vi "TimeSampleDlgModify.vi"(10 "序号":string, 11 "定时采样信息in":T1) -> (2 "定时采样信息":T1)   [LabVIEW 2014, in "Sample.lvlib"]
uses:
  Sample.lvlib
  DataBase/DataBase.lvlib
panel:
  in  "备注":string
  out "电压范围":string
  in  "取消按钮":bool
  in  "确定按钮":bool
  in  "电源频率（Hz）":string="1"
  in  "电源电压":string
  in  "分钟":u16(ring) items=["0", "01", "02", "03", "04", "05", "06", "07", "08", "09", "10", "11", "12", "13", "14", "15", "16", "17", "18", "19", "20", "21", "22", "23", "24", "25", "26", "27", "28", "29", "30", "31", "32", "33", "34", "35", "36", "37", "38", "39", "40", "41", "42", "43", "44", "45", "46", "47", "48", "49", "50", "51", "52", "53", "54", "55", "56", "57", "58", "59"]
  in  "时":u16(ring) items=["1", "2", "3", "4", "5", "6", "7", "8", "9", "10", "11", "12", "13", "14", "15", "16", "17", "18", "19", "20", "21", "22", "23", "24"]
  in  "检测区域":string(combo)
  in  "是否启动":string(combo)="是"
  in  "检测位置":string(combo)="上层膜检测"
  in  "OK":bool
  # "检测时间"
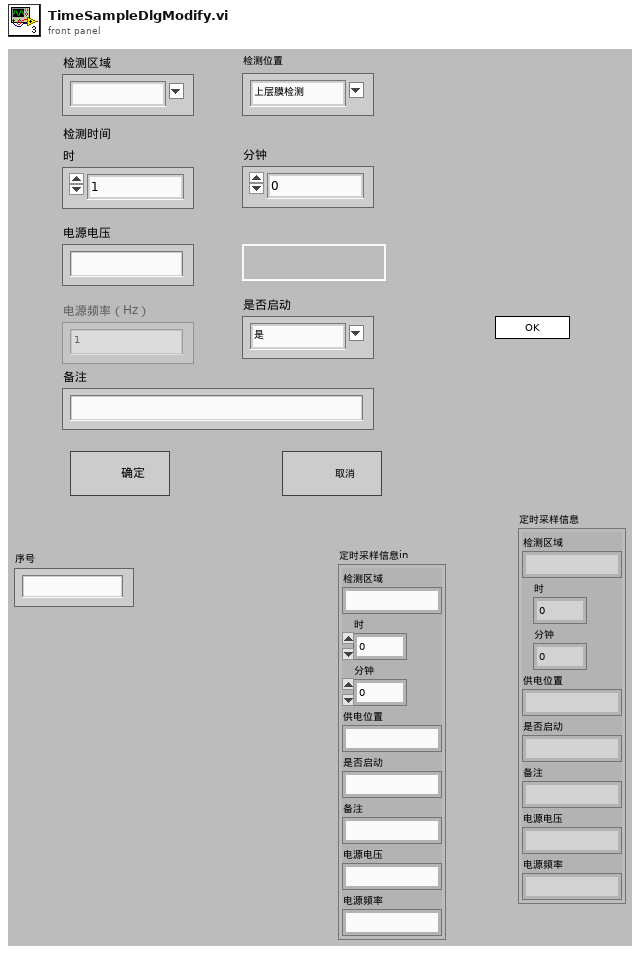
[diagram p1: front panel]
types:
  T1 = cluster{"检测区域":string, "时":u16, "分钟":u16, "供电位置":string, "是否启动":string, "备注":string, "电源电压":string, "电源频率":string}
  T2 = enum32{"invalid app kind", "Development System", "Run Time System", "Student Edition", "Embedded LabVIEW", "Evaluation", "Custom"}
  T3 = enum32{"Invalid", "Standard", "Closed", "Hidden", "Minimized", "Maximized"}
  T4 = cluster{"Core":cluster{"Current VI Reference":refnum<vi>, "Close Panel on Exit?":bool}, "Your Boolean data":bool, "序号":string, "AreaName":string, "SampleAreaName":string[], "定时采样信息":cluster{"检测区域":string, "时":u16, "分钟":u16, "供电位置":string, "是否启动":string, "备注":string, "电源电压":string, "电源频率":string}, "电源倍数":string, "最大电压值":i32, "定时采样info":cluster{"检测区域":string, "时":u16, "分钟":u16, "供电位置":string, "是否启动":string, "备注":string, "电源电压":string, "电源频率":string}}
  T5 = cluster{"Current VI Reference":refnum<vi>, "Close Panel on Exit?":bool}
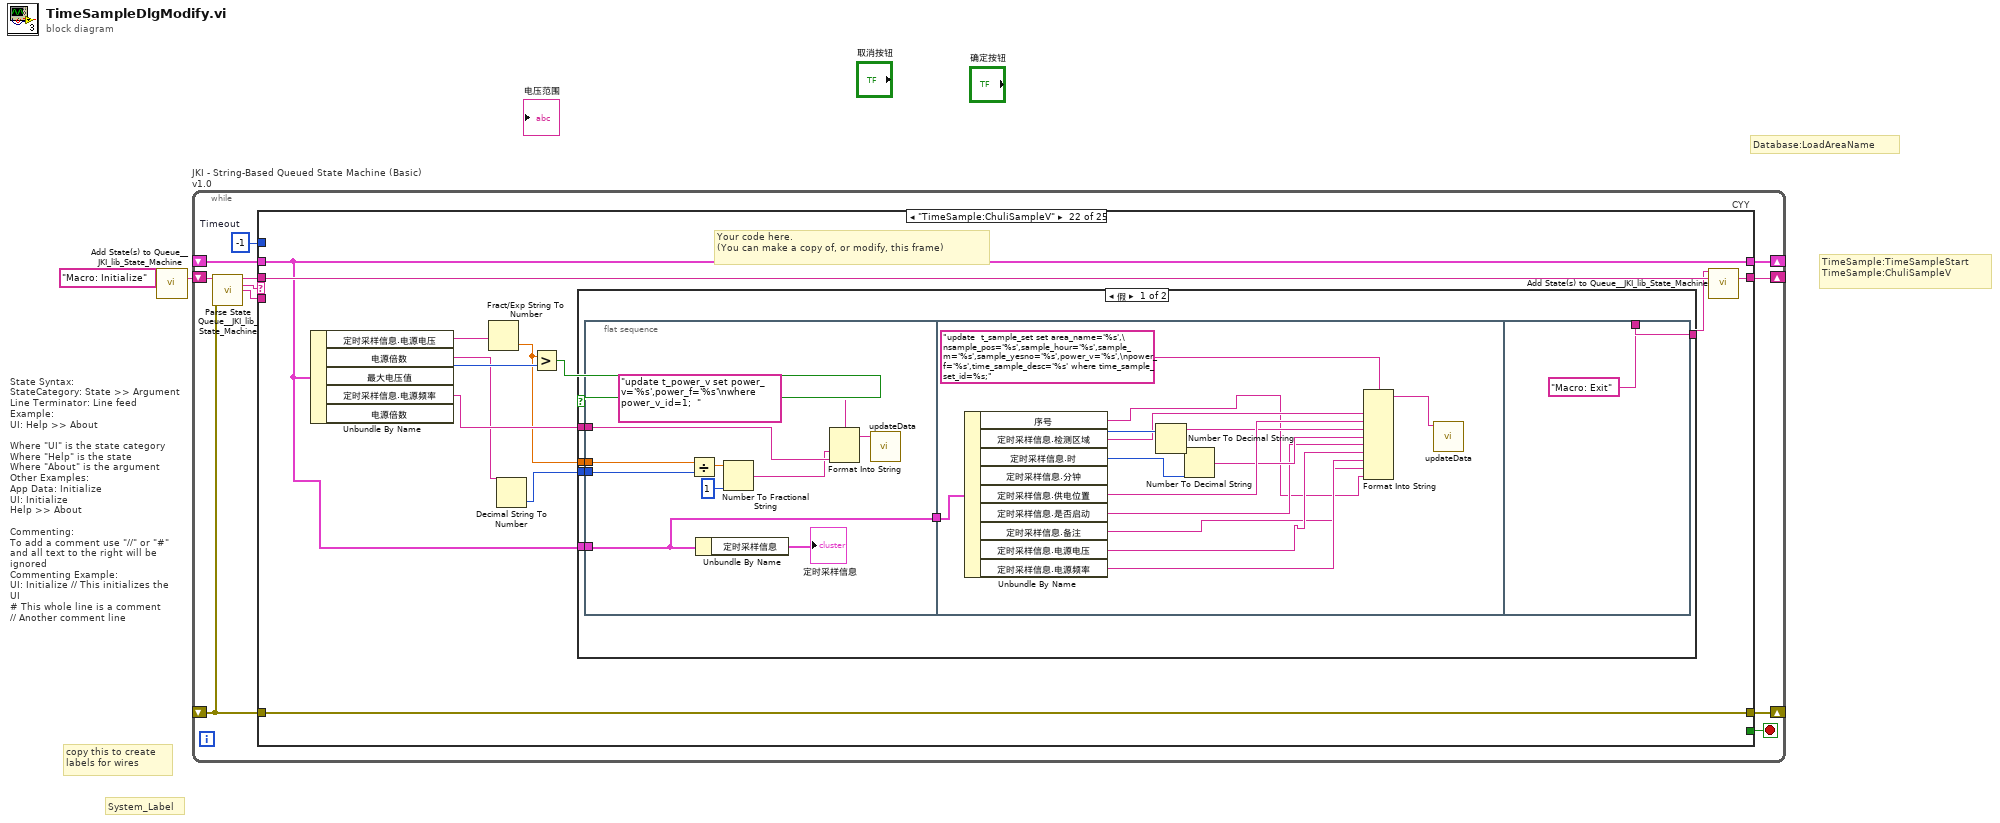
[diagram p0: block diagram]
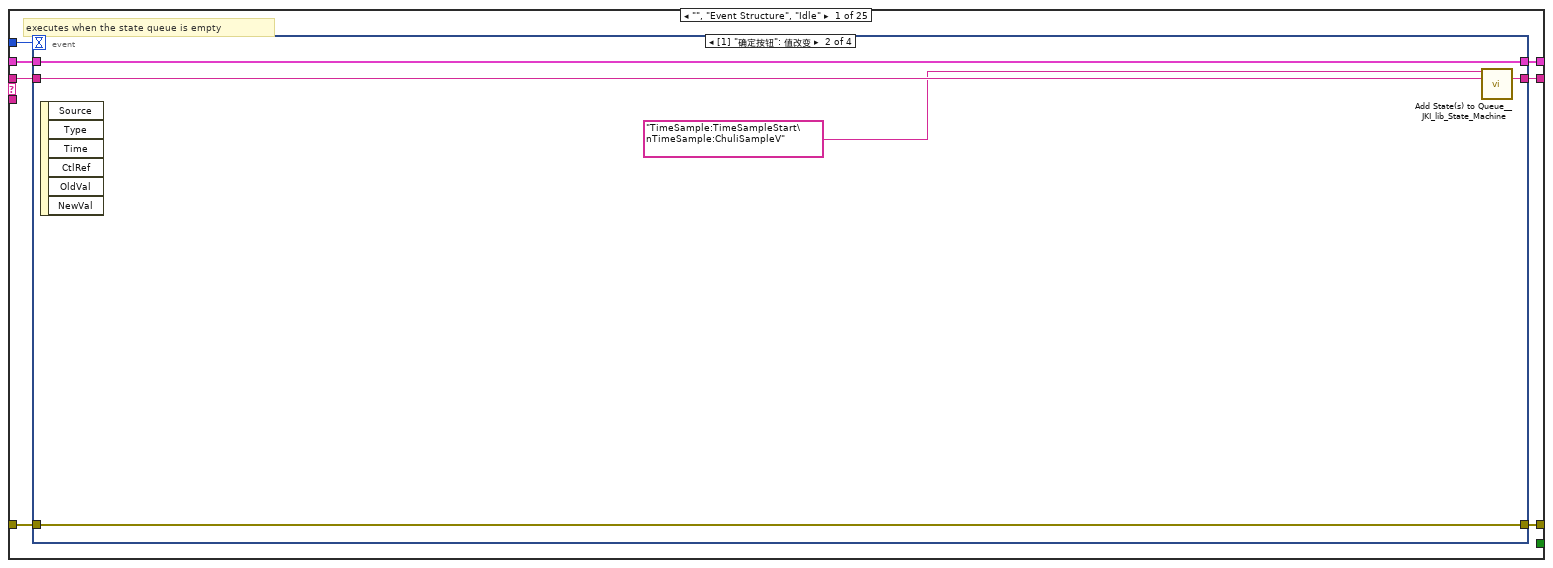
[diagram p2: hidden frame]
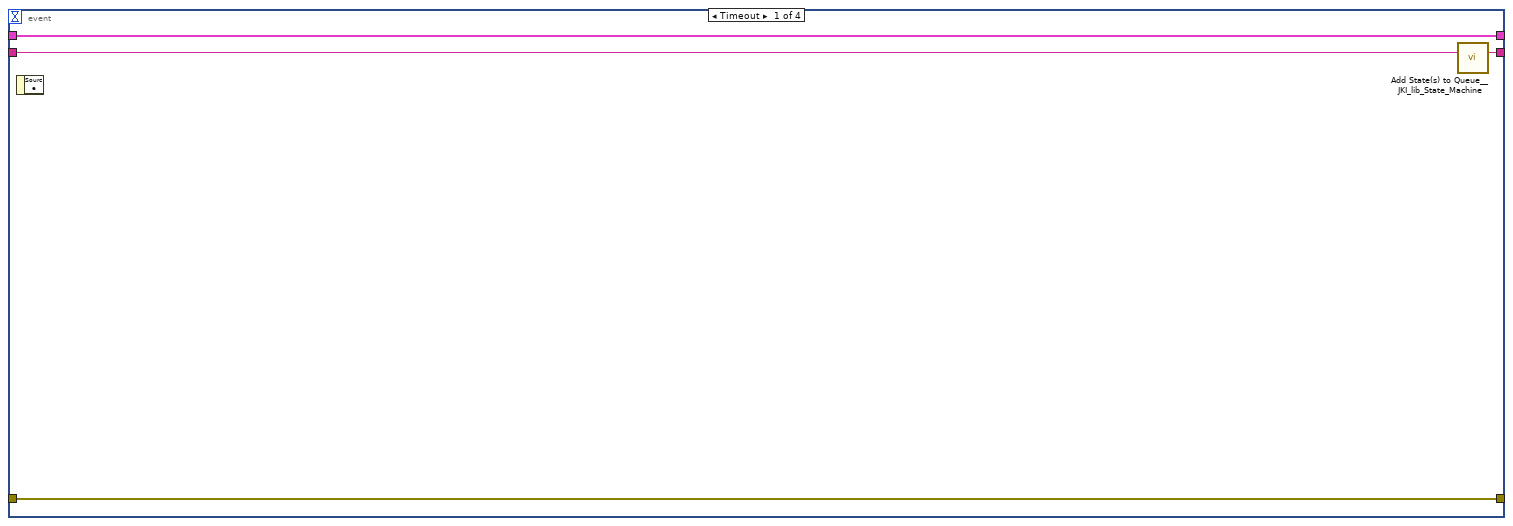
[diagram p3: hidden frame]
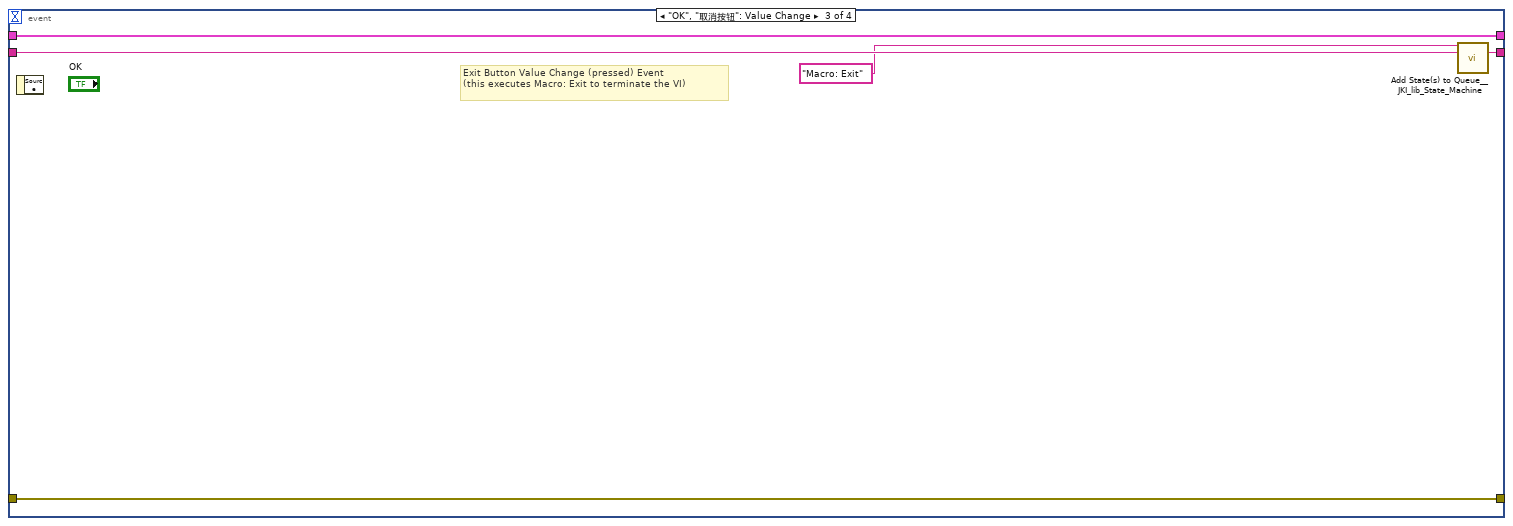
[diagram p4: hidden frame]
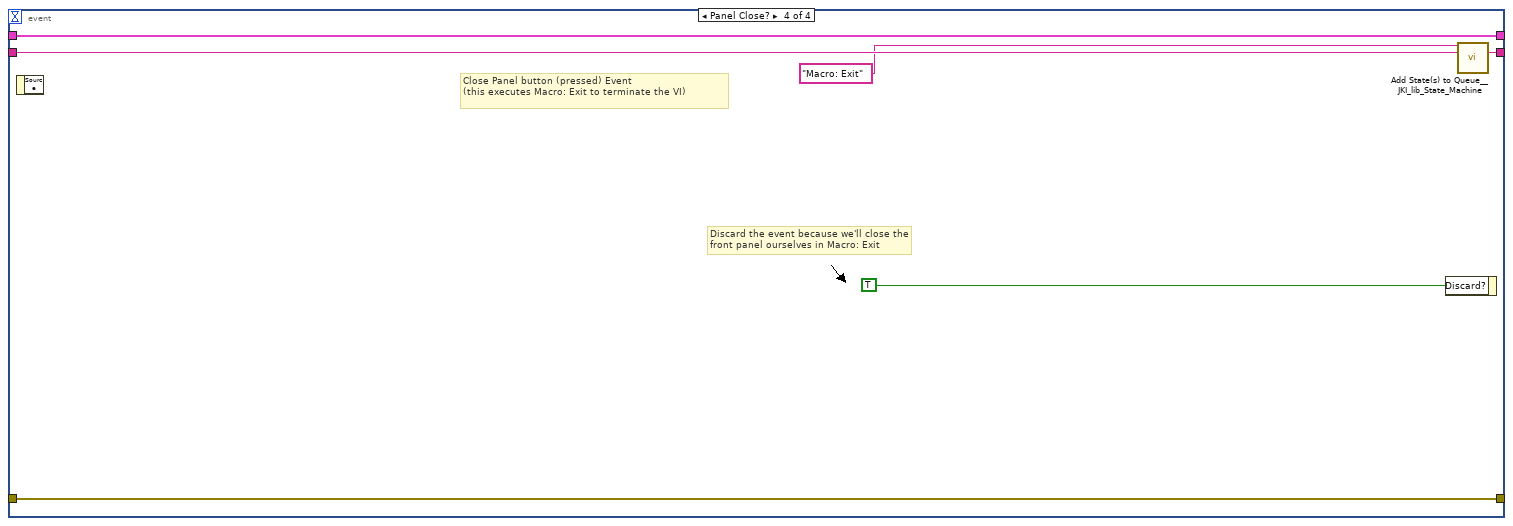
[diagram p5: hidden frame]
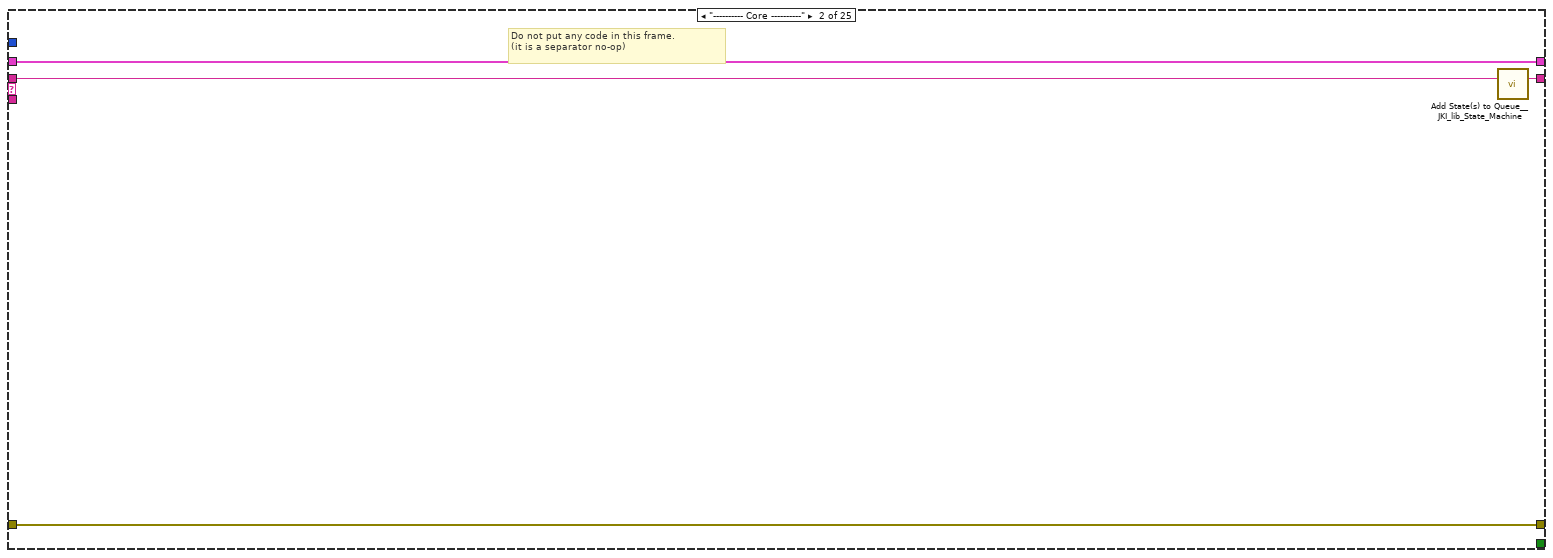
[diagram p6: hidden frame]
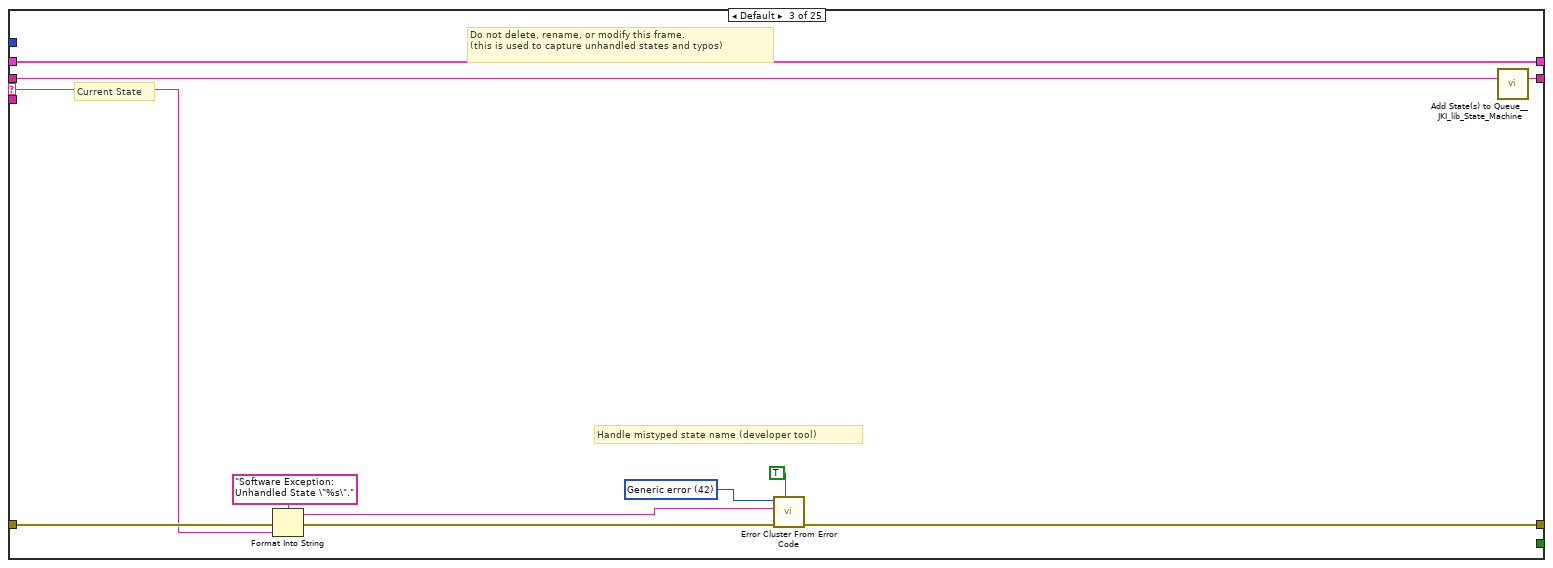
[diagram p7: hidden frame]
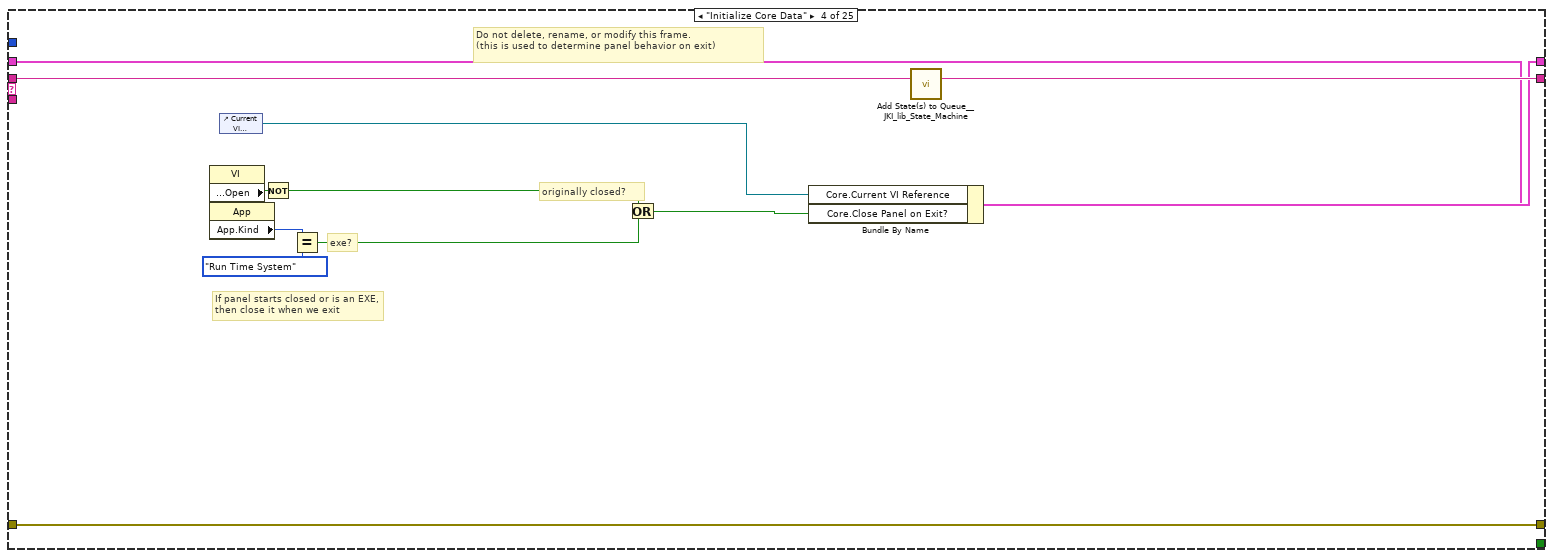
[diagram p8: hidden frame]
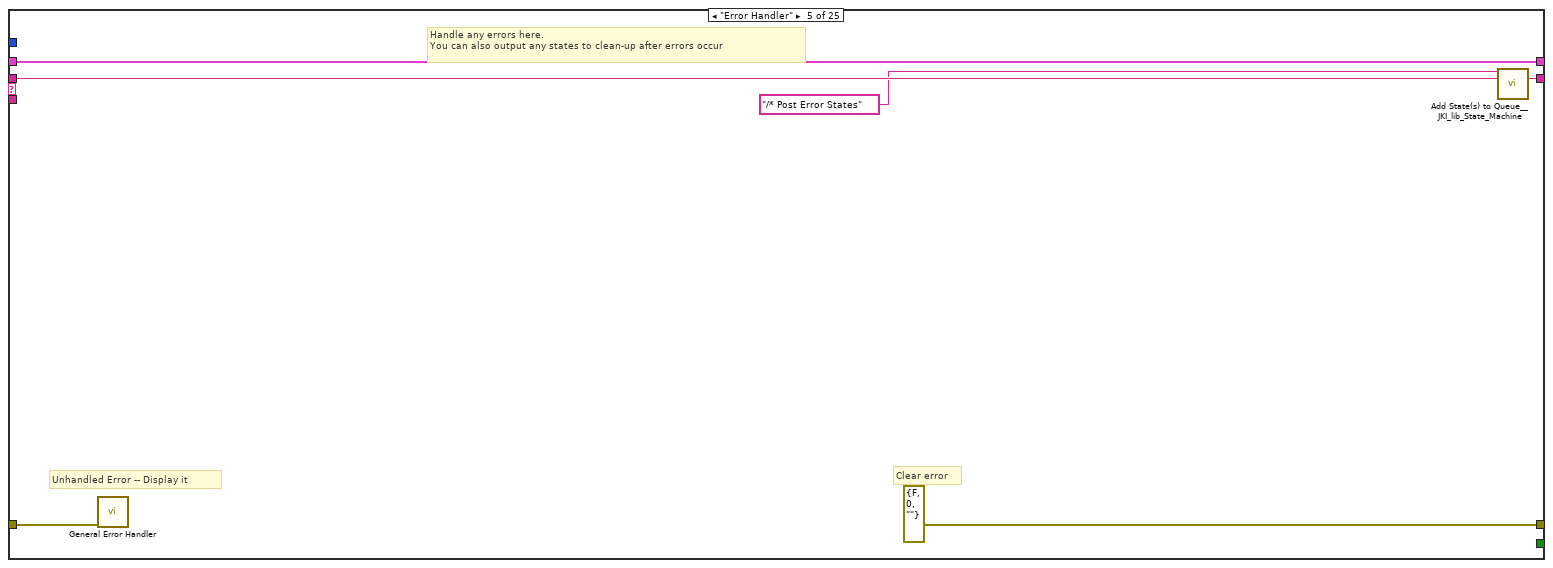
[diagram p9: hidden frame]
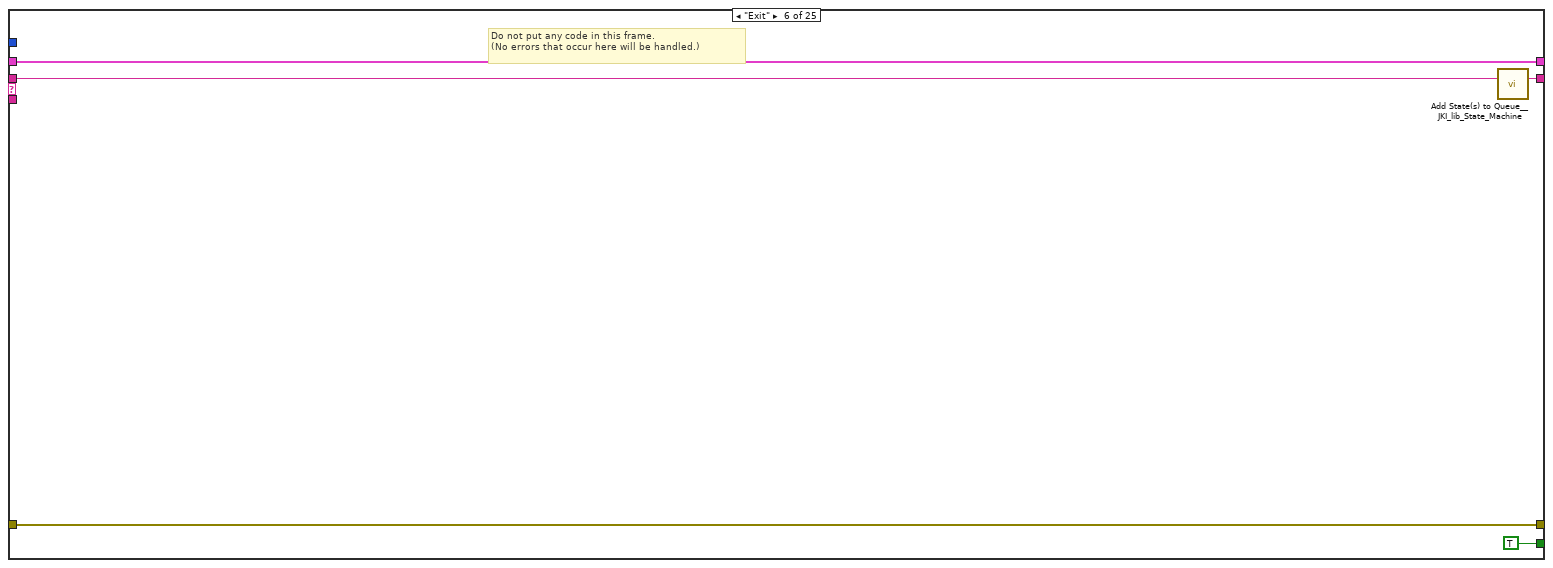
[diagram p10: hidden frame]
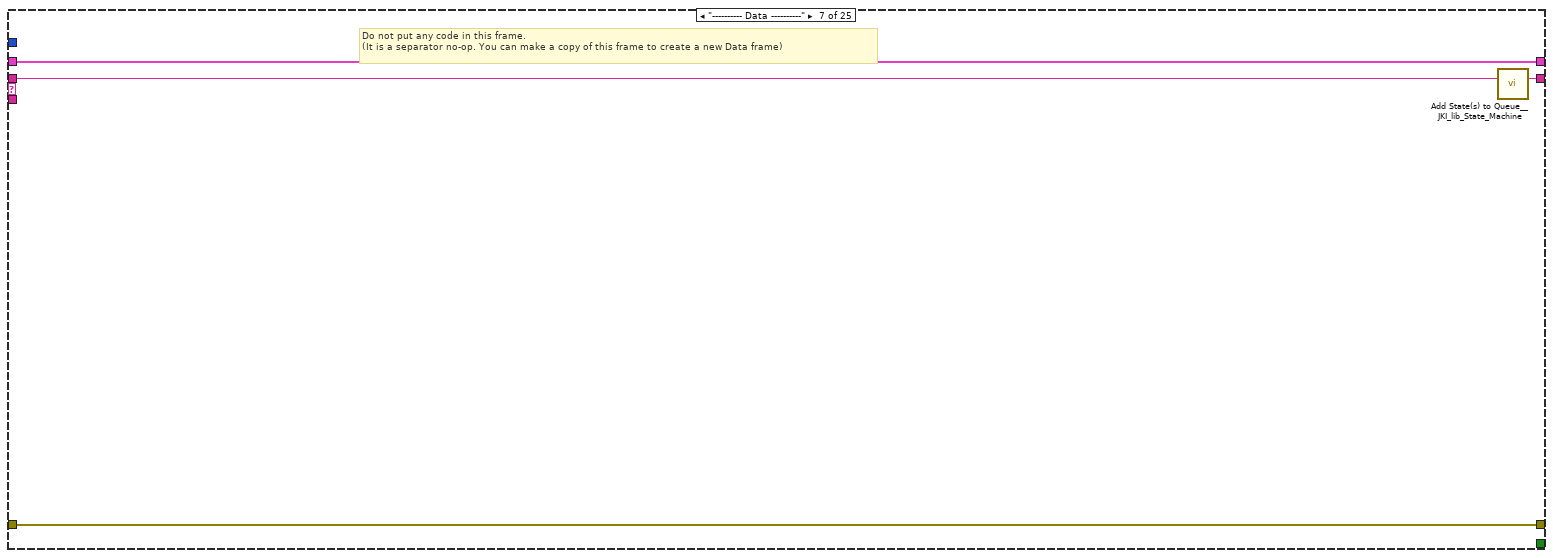
[diagram p11: hidden frame]
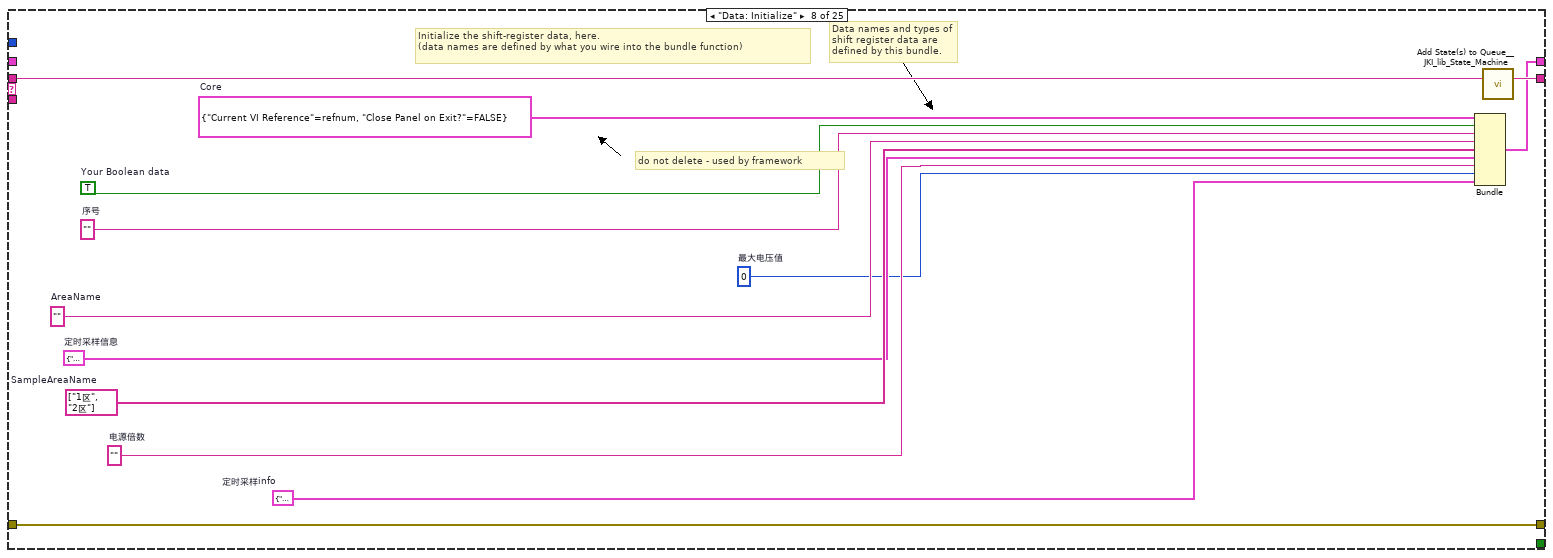
[diagram p12: hidden frame]
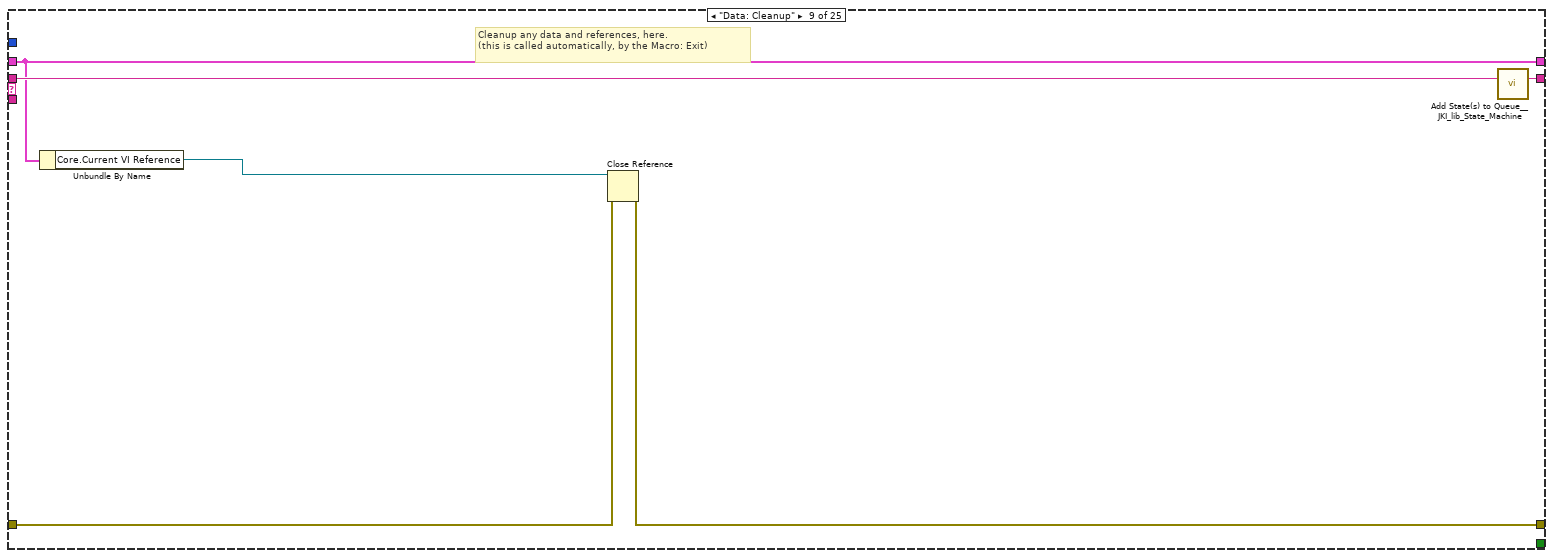
[diagram p13: hidden frame]
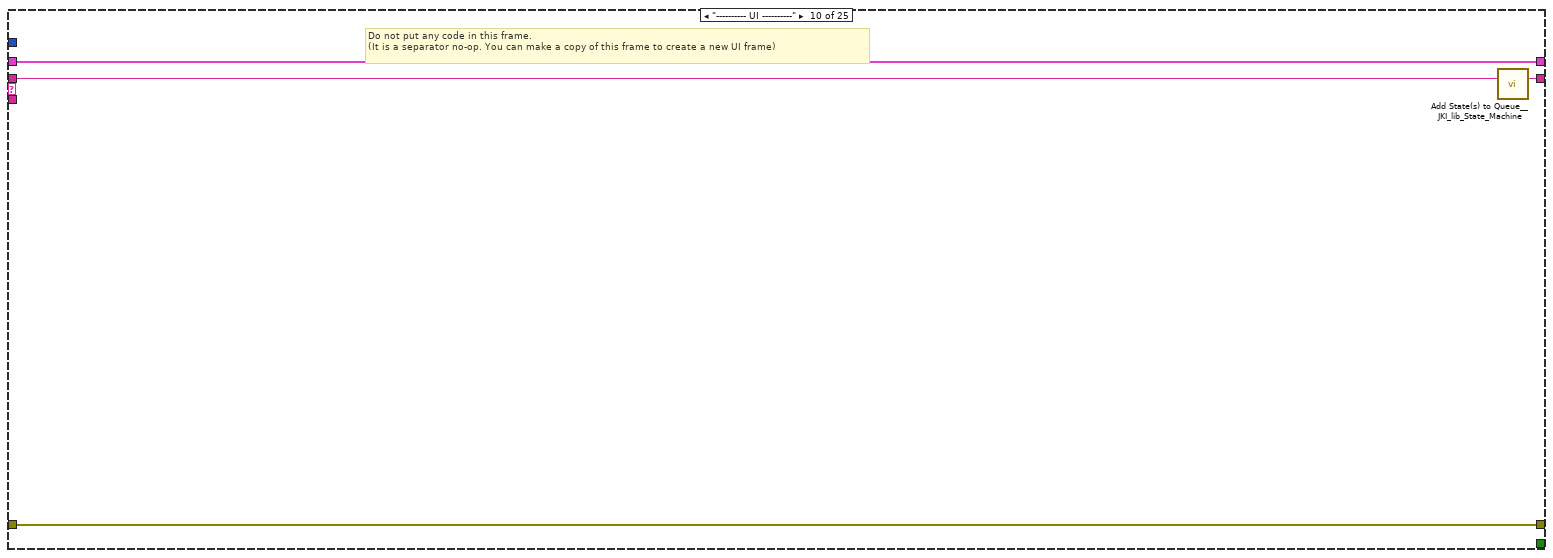
[diagram p14: hidden frame]
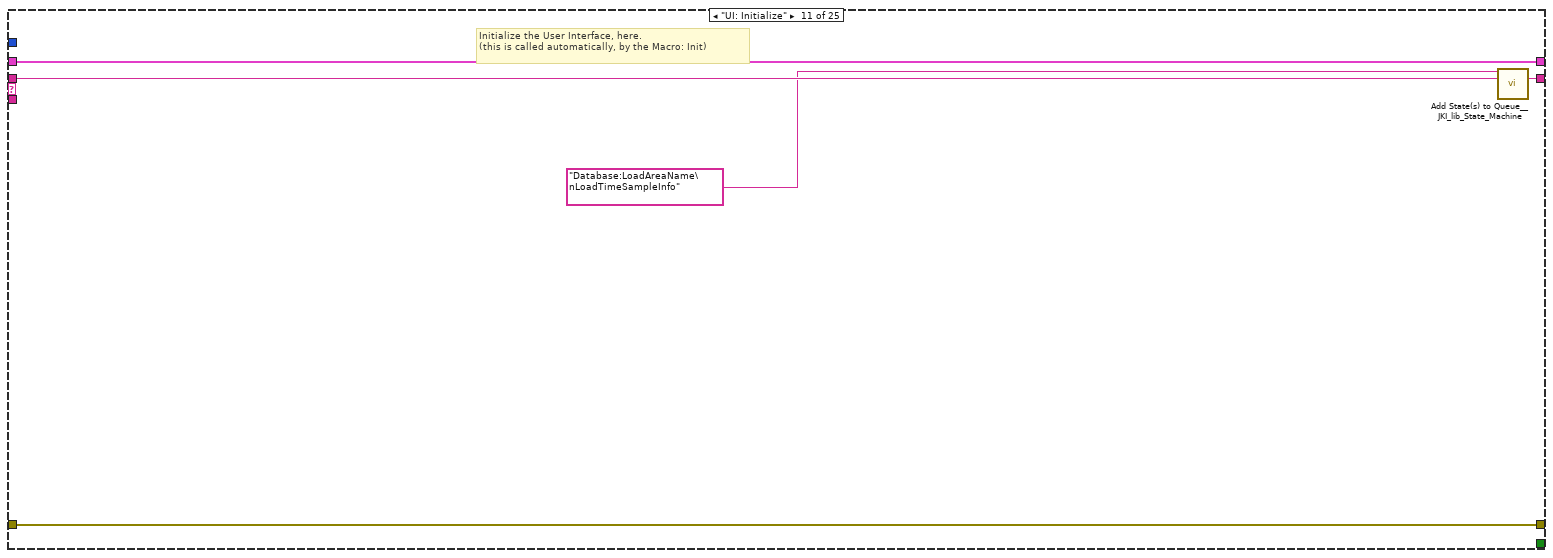
[diagram p15: hidden frame]
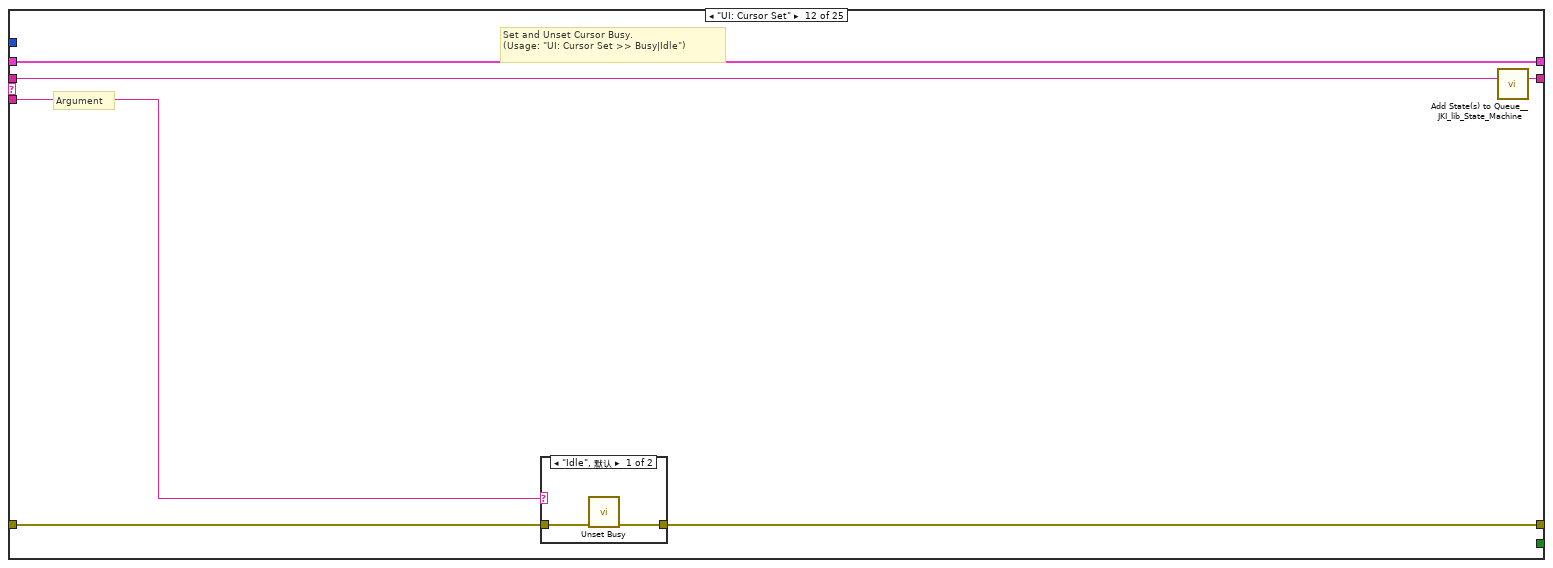
[diagram p16: hidden frame]
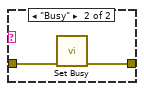
[diagram p17: hidden frame]
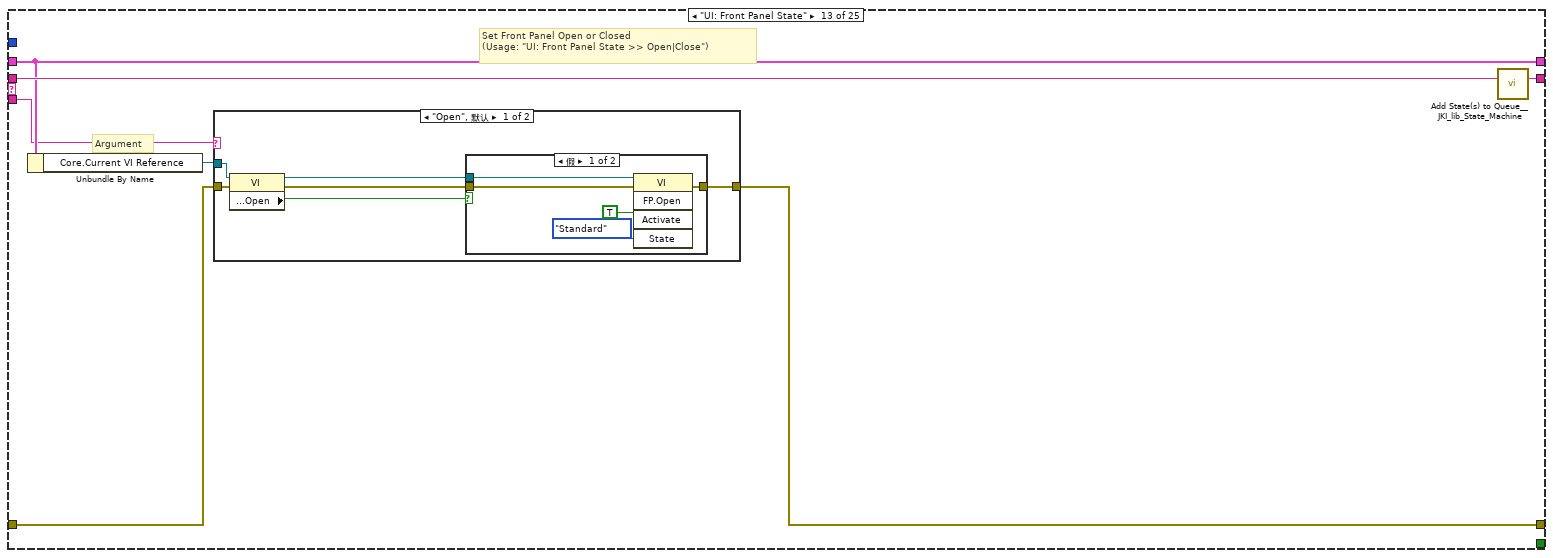
[diagram p18: hidden frame]
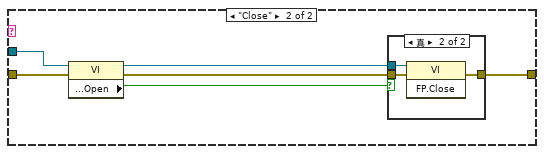
[diagram p20: hidden frame]
diagram:
  # "TimeSample:TimeSampleStart\nTimeSample:ChuliSampleV"
  # "Database:LoadAreaName"
  # "State Syntax:\nStateCategory: State >> Argument\nLine Terminator: Line feed\nExample:\nUI: Help >> About\n\nWhere \"UI\" is the state category\nWhere \"Help\" is the state\nWhere \"About\" is the argument\nOther Examples:\nApp Data: Initialize\nUI: Initialize\nHelp >> About\n\nCommenting:\nTo add a comment use \"//\" or \"#\" and all text to the right will be ignored\nCommenting Example:\nUI: Initialize // This initializes the UI\n# This whole line is a comment\n// Another comment line"
  # "copy this to create labels for wires"
  # "System_Label"
  n1 = call <vilib>:"Add State(s) to Queue__JKI_lib_State_Machine.vi"("State(s) in (\"\")"="Macro: Initialize") -> ("States Out"=w2:string)  [unwired: 14 in]
  n2 = while "JKI - String-Based Queued State Machine (Basic) v1.0" {
    shift-right: [w6] -> _
    shift-left: _ -> [w5]
    shift-right: [w9] -> _
    shift-left: _ -> [w3]
    shift-right: [w8] -> _
    shift-left: w2 -> [w10]
    stop <- w7 stop-if-true
    w4 = -1  # Timeout
    # "CYY"
    n3 = call <vilib>:"Parse State Queue__JKI_lib_State_Machine.vi"("State Queue"=w10, "Error In (no error)"=w3) -> ("Remaining States"=w12:string, "Current State"=w13:string, "Arguments"=w11:string)  [unwired: 11 in]
    n4 = case shown="\"TimeSample:ChuliSampleV\"" w13 {
      selector: w13 -> [_ _ w45 _ _ _ _ _ _ _ _ _ _ _ _ _ _ _ _ _ _ _ _ _ _]
      tunnel: w12 -> [w20 w44 w49 w67 w73 w78 w82 w95 w101 w105 w110 w116 w127 w153 w158 w168 w172 w176 w180 w196 w200 w212 w259 w263 w273]
      tunnel: w11 -> [_ _ _ _ _ _ _ _ _ _ _ w111 w121 _ _ _ _ _ _ _ _ _ _ _ _]
      tunnel: w5 -> [w18 w41 w47 w58 w70 w76 w79 _ w96 w102 w108 w114 w123 w150 w155 w165 w169 w173 w177 w192 w197 w201 w247 w260 w270]
      tunnel: [w17 w42 w51 w64 errorcluster {"status"=FALSE, "code"=0, "source"=""} ("error out") w75 w80 w92 w97 w103 w107 w112 w124 w151 w156 w166 w170 w174 w178 w194 w198 w210 w257 w261 w271] -> w9
      tunnel: w3 -> [w16 w42 w50 w64 w69 w75 w80 w92 w98 w103 w107 w113 w125 w151 w156 w166 w170 w174 w178 w194 w198 w210 w257 w261 w271]
      tunnel: [w19 w43 w48 w66 w72 w77 w81 w94 w100 w104 w109 w115 w126 w152 w157 w167 w171 w175 w179 w195 w199 w211 w258 w262 w272] -> w8
      tunnel: [_ _ _ _ _ TRUE _ _ _ _ _ _ _ _ _ _ _ _ _ _ _ _ _ _ _] -> w7
      tunnel: [w15 w41 w47 w65 w70 w76 w79 w93 w96 w102 w108 w114 w123 w150 w155 w165 w169 w173 w177 w191 w197 w201 w256 w260 w269] -> w6
      tunnel: w4 -> [w14 _ _ _ _ _ _ _ _ _ _ _ _ _ _ _ _ _ _ _ _ _ _ _ _]
      frame "", "Event Structure", "Idle" {
        # "executes when the state queue is empty"
        n5 = event shown="[1] \"确定按钮\": 值改变" {
          selector: _ -> [_ _ _ _]
          dyn-events: _ -> [_ _ _ _]
          timeout: w14 -> [_ _ _ _]
          tunnel: w20 -> [w24 w29 w34 w40]
          tunnel: [w23 w28 w33 w39] -> w19
          tunnel: w18 -> [w21 w26 w31 w37]
          tunnel: [w22 w27 w32 w38] -> w17
          tunnel: w16 -> [w22 w27 w32 w38]
          tunnel: [w21 w26 w31 w37] -> w15
          event Timeout {
            n6 = event-data() -> ()  [unwired: 1 in, 1 out]
            n7 = call <vilib>:"Add State(s) to Queue__JKI_lib_State_Machine.vi"("State(s) in (\"\")"=w24) -> ("States Out"=w23:string)  [unwired: 14 in]
          }
          event "确定按钮": Value Change {
            n8 = event-data() -> ()  [unwired: 1 in, 6 out]
            n9 = call <vilib>:"Add State(s) to Queue__JKI_lib_State_Machine.vi"("State(s) in Front (\"\")"="TimeSample:TimeSampleStart\nTimeSample:ChuliSampleV", "State(s) in (\"\")"=w29) -> ("States Out"=w28:string)  [unwired: 13 in]
          }
          event "OK", "取消按钮": Value Change {
            # "Exit Button Value Change (pressed) Event\n(this executes Macro: Exit to terminate the VI)"
            n10 = event-data() -> ()  [unwired: 1 in, 1 out]
            n11 = call <vilib>:"Add State(s) to Queue__JKI_lib_State_Machine.vi"("State(s) in Front (\"\")"="Macro: Exit", "State(s) in (\"\")"=w34) -> ("States Out"=w33:string)  [unwired: 13 in]
          }
          event Panel Close? {
            # "Discard the event because we'll close the front panel ourselves in Macro: Exit"
            # "Close Panel button (pressed) Event\n(this executes Macro: Exit to terminate the VI)"
            n12 = event-data() -> ()  [unwired: 1 in, 1 out]
            n13 = event-data("Discard?"=TRUE) -> ()  [unwired: 1 in, 1 out]
            n14 = call <vilib>:"Add State(s) to Queue__JKI_lib_State_Machine.vi"("State(s) in Front (\"\")"="Macro: Exit", "State(s) in (\"\")"=w40) -> ("States Out"=w39:string)  [unwired: 13 in]
          }
        }
      }
      frame "---------- Core ----------" {
        # "Do not put any code in this frame.\n(it is a separator no-op)"
        n15 = call <vilib>:"Add State(s) to Queue__JKI_lib_State_Machine.vi"("State(s) in (\"\")"=w44) -> ("States Out"=w43:string)  [unwired: 14 in]
      }
      frame Default {
        w54 = 42 items=["No error", "Argument error", "Memory is full", "Out of zone", "End of file", "File already open", "Generic file I/O error", "File not found", "File permission error", "Disk is full", "Duplicate path", "Too many files open", "System feature not enabled", "Resource file not found", "Cannot add resource", "Resource not found", "Image not found", "Image memory error", "Pen does not exist", "Config type invalid", "Config token not found", "Config parse error", "Config memory error", "Bad external code format", "Bad external code offset", "External code not present", "Null window", "Destroy window error", "Null menu", "Print aborted", "Bad print record", "Print driver error", "Windows error during printing", "Memory error during printing", "Print dialog error", "Generic print error", "Invalid device refnum", "Device not found", "Device parameter error", "Device unit error", "Cannot open device", "Device call aborted", "Generic error", "Cancelled by user", "Object ID too low", "Object ID too high", "Object not in heap", "Unknown heap", "Unknown object (invalid DefProc)", "Unknown object (DefProc not in table)", "Message out of range", "Invalid (null) method", "Unknown message", "Manager call not supported", "Bad address", "Network operation in progress", "Network operation timed out", "Connection is busy", "Network attribute not supported", "Network error", "Address in use", "System out of memory", "Connection aborted", "Connection refused", "Not connected", "Already connected", "Connection closed", "Initialization error (interapplication manager)", "Bad occurrence", "Wait on unbound occurrence handler", "Occurrence queue overflow", "Datalog type conflict", "Unused", "Unrecognized type (interapplication manager)", "Memory corrupt", "Failed to make temporary DLL", "Old CIN version", "Drag socket not found", "Failed to load drop-object", "Failed to register OLE object", "Failed to release OLE object", "Format specifier type mismatch", "Unknown format specifier", "Too few format specifiers", "Too many format specifiers", "Scan failed", "Newer CIN version", "Error converting to variant", "Runtime menu error", "Password tampered", "Variant attribute not found", "Incompatible variant data type", "Event data is not available", "Event Store is not present", "Occurrence is not found", "Event Queue is not created", "Event info is not available", "Refnum passed is NULL", "Error retrieving Class GUID", "Error retrieving CoClass GUID", "Error retrieving TypeLib GUID.", "Bad built application magic bytes.", "Specific driver is different from the specific driver associated with the Logical Name.", "There is no session opened to the class driver.", "Max Error", "MAX - Error with config objects", "MAX - Error loading configuration", "MAX - Group not supported"]
        # "Current State"
        # "Do not delete, rename, or modify this frame.\n(this is used to capture unhandled states and typos)"
        # "Handle mistyped state name (developer tool)"
        n16 = Format Into String(format string="Software Exception: Unhandled State \"%s\"." ("message"), error in=w50, w45) -> (resulting string=w53:string, error out=w52:errorcluster)  [unwired: 1 in]
        n17 = call <vilib>:"Error Cluster From Error Code.vi"("show call chain? (False)"=TRUE, "error in (no error)"=w52, "error message (\"\")"=w53, "error code (0)"=w54) -> ("error out"=w51:errorcluster)  [unwired: 5 in]
        n18 = call <vilib>:"Add State(s) to Queue__JKI_lib_State_Machine.vi"("State(s) in (\"\")"=w49) -> ("States Out"=w48:string)  [unwired: 14 in]
      }
      frame "Initialize Core Data" {
        # "Do not delete, rename, or modify this frame.\n(this is used to determine panel behavior on exit)"
        # "originally closed?"
        # "exe?"
        # "If panel starts closed or is an EXE, then close it when we exit"
        n19 = property class="VI"() -> ("Front Panel.Open"=w63:bool)  [unwired: 2 in, 2 out]
        n20 = property class="App"() -> ("App.Kind"=w62:T2)  [unwired: 2 in, 2 out]
        n21 = control-ref of="Current VI Reference"() -> (w56:refnum<vi>)
        n22 = Not(x=w63) -> (.not. x?=w60:bool)
        n23 = Equal?(x=w62, y=T2."Run Time System" ("Application:Kind")) -> (x = y?=w59:bool)
        n24 = Or(x=w60, y=w59) -> (x .or. y?=w57:bool)
        n25 = Bundle By Name(cluster=w58, "Core.Current VI Reference"=w56, "Core.Close Panel on Exit?"=w57) -> (w65:T4)
        n26 = call <vilib>:"Add State(s) to Queue__JKI_lib_State_Machine.vi"("State(s) in (\"\")"=w67) -> ("States Out"=w66:string)  [unwired: 14 in]
      }
      frame "Error Handler" {
        # "Unhandled Error -- Display it"
        # "Handle any errors here.\nYou can also output any states to clean-up after errors occur"
        # "Clear error"
        n27 = call <vilib>:"General Error Handler.vi"("error in (no error)"=w69) -> ()  [unwired: 10 in, 5 out]
        n28 = call <vilib>:"Add State(s) to Queue__JKI_lib_State_Machine.vi"("State(s) in Front (\"\")"="/* Post Error States", "State(s) in (\"\")"=w73) -> ("States Out"=w72:string)  [unwired: 13 in]
      }
      frame "Exit" {
        # "Do not put any code in this frame.\n(No errors that occur here will be handled.)"
        n29 = call <vilib>:"Add State(s) to Queue__JKI_lib_State_Machine.vi"("State(s) in (\"\")"=w78) -> ("States Out"=w77:string)  [unwired: 14 in]
      }
      frame "---------- Data ----------" {
        # "Do not put any code in this frame.\n(It is a separator no-op. You can make a copy of this frame to create a new Data frame)"
        n30 = call <vilib>:"Add State(s) to Queue__JKI_lib_State_Machine.vi"("State(s) in (\"\")"=w82) -> ("States Out"=w81:string)  [unwired: 14 in]
      }
      frame "Data: Initialize" {
        w83 = T1 {"检测区域"="", "时"=0, "分钟"=0, "供电位置"="", "是否启动"="", "备注"="", "电源电压"="", "电源频率"=""}  # 定时采样info
        w84 = 0  # 最大电压值
        w85 = ""  # 电源倍数
        w86 = T1 {"检测区域"="", "时"=0, "分钟"=0, "供电位置"="", "是否启动"="", "备注"="", "电源电压"="", "电源频率"=""}  # 定时采样信息
        w87 = string[] ["1区", "2区"]  # SampleAreaName
        w88 = ""  # AreaName
        w89 = T5 {"Current VI Reference"=refnum, "Close Panel on Exit?"=FALSE}  # Core
        w91 = TRUE  # Your Boolean data
        w90 = ""  # 序号
        # "do not delete - used by framework"
        # "Data names and types of shift register data are defined by this bundle."
        # "Initialize the shift-register data, here.\n(data names are defined by what you wire into the bundle function)"
        n31 = Bundle("Core"=w89, "Your Boolean data"=w91, "序号"=w90, "AreaName"=w88, "SampleAreaName"=w87, "定时采样信息"=w86, "电源倍数"=w85, "最大电压值"=w84, "定时采样info"=w83) -> (w93:T4)  [unwired: 1 in]
        n32 = call <vilib>:"Add State(s) to Queue__JKI_lib_State_Machine.vi"("State(s) in (\"\")"=w95) -> ("States Out"=w94:string)  [unwired: 14 in]
      }
      frame "Data: Cleanup" {
        # "Cleanup any data and references, here.\n(this is called automatically, by the Macro: Exit)"
        n33 = Unbundle By Name(w96) -> ("Core.Current VI Reference"=w99:refnum<vi>)
        n34 = Close Reference(reference=w99, error in (no error)=w98) -> (error out=w97:errorcluster)
        n35 = call <vilib>:"Add State(s) to Queue__JKI_lib_State_Machine.vi"("State(s) in (\"\")"=w101) -> ("States Out"=w100:string)  [unwired: 14 in]
      }
      frame "---------- UI ----------" {
        # "Do not put any code in this frame.\n(It is a separator no-op. You can make a copy of this frame to create a new UI frame)"
        n36 = call <vilib>:"Add State(s) to Queue__JKI_lib_State_Machine.vi"("State(s) in (\"\")"=w105) -> ("States Out"=w104:string)  [unwired: 14 in]
      }
      frame "UI: Initialize" {
        # "Initialize the User Interface, here.\n(this is called automatically, by the Macro: Init)"
        n37 = call <vilib>:"Add State(s) to Queue__JKI_lib_State_Machine.vi"("State(s) in Front (\"\")"="Database:LoadAreaName\nLoadTimeSampleInfo", "State(s) in (\"\")"=w110) -> ("States Out"=w109:string)  [unwired: 13 in]
      }
      frame "UI: Cursor Set" {
        # "Argument"
        # "Set and Unset Cursor Busy.\n(Usage: \"UI: Cursor Set >> Busy|Idle\")"
        n38 = case shown="\"Idle\", 默认" w111 {
          tunnel: w113 -> [w118 w120]
          tunnel: [w117 w119] -> w112
          frame "Idle", Default {
            n39 = call <vilib>:"Unset Busy.vi"("error in (no error)"=w118) -> ("error out"=w117:errorcluster)  [unwired: 10 in]
          }
          frame "Busy" {
            n40 = call <vilib>:"Set Busy.vi"("error in (no error)"=w120) -> ("error out"=w119:errorcluster)  [unwired: 9 in, 1 out]
          }
        }
        n41 = call <vilib>:"Add State(s) to Queue__JKI_lib_State_Machine.vi"("State(s) in (\"\")"=w116) -> ("States Out"=w115:string)  [unwired: 14 in]
      }
      frame "UI: Front Panel State" {
        # "Argument"
        # "Set Front Panel Open or Closed\n(Usage: \"UI: Front Panel State >> Open|Close\")"
        n42 = Unbundle By Name(w123) -> ("Core.Current VI Reference"=w122:refnum<vi>)
        n43 = case shown="\"Open\", 默认" w121 {
          tunnel: w125 -> [w131 w144]
          tunnel: [w133 w145] -> w124
          tunnel: w122 -> [w132 w142]
          frame "Open", Default {
            n44 = property class="VI"(reference=w132, error in=w131) -> (reference out=w129:refnum<vi>, error out=w130:errorcluster, "Front Panel.Open"=w128:bool)
            n45 = case shown="假" w128 {
              tunnel: [w136 w139] -> w133
              tunnel: w130 -> [w135 w139]
              tunnel: w129 -> [w134 _]
              frame False {
                n46 = invoke class="VI" method="FP.Open"(reference=w134, error in=w135, "Activate"=TRUE, "State"=T3."Standard") -> (error out=w136:errorcluster)  [unwired: 1 in, 4 out]
              }
              frame True {
              }
            }
          }
          frame "Close" {
            n47 = property class="VI"(reference=w142, error in=w144) -> (reference out=w141:refnum<vi>, error out=w143:errorcluster, "Front Panel.Open"=w140:bool)
            n48 = case shown="真" w140 {
              tunnel: [w146 w149] -> w145
              tunnel: w143 -> [w146 w148]
              tunnel: w141 -> [_ w147]
              frame False {
              }
              frame True {
                n49 = invoke class="VI" method="FP.Close"(reference=w147, error in=w148) -> (error out=w149:errorcluster)  [unwired: 1 in, 2 out]
              }
            }
          }
        }
        n50 = call <vilib>:"Add State(s) to Queue__JKI_lib_State_Machine.vi"("State(s) in (\"\")"=w127) -> ("States Out"=w126:string)  [unwired: 14 in]
      }
      frame "---------- Macro ----------" {
        # "Do not put any code in this frame.\n(It is a separator no-op. You can make a copy of this frame to create a new Macro frame)"
        n51 = call <vilib>:"Add State(s) to Queue__JKI_lib_State_Machine.vi"("State(s) in (\"\")"=w153) -> ("States Out"=w152:string)  [unwired: 14 in]
      }
      frame "Macro: Initialize" {
        w154 = "Data: Initialize\nInitialize Core Data\nUI: Initialize\nUI: Front Panel State >> Open"  # Data: Initialize Initialize Core Data UI: Initialize UI: Front Panel State >> Open
        # "Initialization Macro\n(This is called once, when the VI starts)"
        n52 = call <vilib>:"Add State(s) to Queue__JKI_lib_State_Machine.vi"("State(s) in Front (\"\")"=w154, "State(s) in (\"\")"=w158) -> ("States Out"=w157:string)  [unwired: 13 in]
      }
      frame "Macro: Exit" {
        # "Exit Macro\n(This is called once, when the VI exits)"
        n53 = Unbundle By Name(w165) -> ("Core.Close Panel on Exit?"=w164:bool)
        n54 = Select(t="UI: Front Panel State >> Close", s=w164, f="") -> (s? t:f=w161:string)
        n55 = call <vilib>:"Add State(s) to Queue__JKI_lib_State_Machine.vi"("State(s) in (\"\")"=w161, "State(s) at Back (\"\")"="Data: Cleanup\nExit") -> ("States Out"=w159:string)  [unwired: 13 in]
        n56 = call <vilib>:"Add State(s) to Queue__JKI_lib_State_Machine.vi"("State(s) in Front (\"\")"=w159, "State(s) in (\"\")"=w168) -> ("States Out"=w167:string)  [unwired: 13 in]
      }
      frame "---------- New Category ----------" {
        # "Template Separator\n(You can make a copy of, or modify, this frame)"
        n57 = call <vilib>:"Add State(s) to Queue__JKI_lib_State_Machine.vi"("State(s) in (\"\")"=w172) -> ("States Out"=w171:string)  [unwired: 14 in]
      }
      frame "New Category: 1" {
        # "Your code here.\n(You can make a copy of, or modify, this frame)"
        n58 = call <vilib>:"Add State(s) to Queue__JKI_lib_State_Machine.vi"("State(s) in (\"\")"=w176) -> ("States Out"=w175:string)  [unwired: 14 in]
      }
      frame "New Category: 2" {
        # "Your code here.\n(You can make a copy of, or modify, this frame)"
        n59 = call <vilib>:"Add State(s) to Queue__JKI_lib_State_Machine.vi"("State(s) in (\"\")"=w180) -> ("States Out"=w179:string)  [unwired: 14 in]
      }
      frame "LoadTimeSampleInfo" {
        # "Your code here.\n(You can make a copy of, or modify, this frame)"
        n60 = Bundle By Name(cluster=w192, "定时采样info"="定时采样信息in", "序号"="序号") -> (w191:T4)
        n61 = Unbundle By Name(w191) -> ("定时采样info.检测区域"=w189:string, "定时采样info.时"=w182:u16, "定时采样info.分钟"=w188:u16, "定时采样info.供电位置"=w187:string, "定时采样info.是否启动"=w186:string, "定时采样info.备注"=w185:string, "定时采样info.电源电压"=w190:string, "定时采样info.电源频率"=w184:string)
        n62 = Decrement(x=w182) -> (x-1=w181:u16)
        n63 = local write "电源电压"(w190) -> ()
        n64 = local write "时"(w181) -> ()
        n65 = local write "检测区域"(w189) -> ()
        n66 = local write "检测位置"(w187) -> ()
        n67 = local write "电源频率（Hz）"(w184) -> ()
        n68 = local write "分钟"(w188) -> ()
        n69 = local write "是否启动"(w186) -> ()
        n70 = local write "备注"(w185) -> ()
        n71 = call <vilib>:"Add State(s) to Queue__JKI_lib_State_Machine.vi"("State(s) in (\"\")"=w196) -> ("States Out"=w195:string)  [unwired: 14 in]
      }
      frame "---------TimeSample--------" {
        # "Your code here.\n(You can make a copy of, or modify, this frame)"
        n72 = call <vilib>:"Add State(s) to Queue__JKI_lib_State_Machine.vi"("State(s) in (\"\")"=w200) -> ("States Out"=w199:string)  [unwired: 14 in]
      }
      frame "TimeSample:ChuliSampleV" {
        # "Your code here.\n(You can make a copy of, or modify, this frame)"
        n73 = Unbundle By Name(w201) -> ("定时采样信息.电源电压"=w209:string, "电源倍数"=w203:string, "最大电压值"=w208:i32, "定时采样信息.电源频率"=w205:string)  [unwired: 1 out]
        n74 = Fract/Exp String To Number(string=w209) -> (number=w204:dbl)  [unwired: 3 in, 1 out]
        n75 = Decimal String To Number(string=w203) -> (number=w202:i32)  [unwired: 2 in, 1 out]
        n76 = Greater?(x=w204, y=w208) -> (0:w207:bool)
        n77 = case shown="假" w207 {
          tunnel: [w214 ""] -> w206
          tunnel: w205 -> [w218 _]
          tunnel: w204 -> [w217 _]
          tunnel: w202 -> [w216 _]
          tunnel: w201 -> [w215 _]
          frame False {
            n78 = flat-sequence {
              tunnel: w218 -> [w226]
              tunnel: w217 -> [w223]
              tunnel: w216 -> [w222]
              tunnel: w215 -> [w219]
              tunnel: [w219] -> w213
              tunnel: w213 -> [w242]
              tunnel: ["Macro: Exit"] -> w214
              frame #0 {
                n79 = Divide(x=w223, y=w222) -> (x/y=w225:dbl)
                n80 = Unbundle By Name(w219) -> ("定时采样信息"=→"定时采样信息":T1)
                n81 = Number To Fractional String(number=w225, precision (6)=i16 1 ("精度(6)")) -> (F-format string=w221:string)  [unwired: 2 in]
                n82 = Format Into String(format string="update t_power_v set power_v='%s',power_f='%s'\nwhere power_v_id=1;  ", w221, w226) -> (resulting string=w228:string)  [unwired: 2 in, 1 out]
                n83 = call "updateData.vi"("SQL query"=w228) -> ()  [unwired: 10 in, 1 out]
              }
              frame #1 {
                n84 = Unbundle By Name(w242) -> ("序号"=w230:string, "定时采样信息.检测区域"=w238:string, "定时采样信息.时"=w241:u16, "定时采样信息.分钟"=w240:u16, "定时采样信息.供电位置"=w237:string, "定时采样信息.是否启动"=w234:string, "定时采样信息.备注"=w231:string, "定时采样信息.电源电压"=w233:string, "定时采样信息.电源频率"=w232:string)
                n85 = Number To Decimal String(number=w241) -> (decimal integer string=w236:string)  [unwired: 1 in]
                n86 = Number To Decimal String(number=w240) -> (decimal integer string=w235:string)  [unwired: 1 in]
                n87 = Format Into String(format string="update  t_sample_set set area_name='%s',\nsample_pos='%s',sample_hour='%s',sample_m='%s',sample_yesno='%s',power_v='%s',\npower_f='%s',time_sample_desc='%s' where time_sample_set_id=%s;", w238, w237, w236, w235, w234, w233, w232, w231, w230) -> (resulting string=w229:string)  [unwired: 2 in, 1 out]
                n88 = call "updateData.vi"("SQL query"=w229) -> ()  [unwired: 10 in, 1 out]
              }
              frame #2 {
              }
            }
          }
          frame True {
            n89 = One Button Dialog(message="电压超过范围，请从新输入") -> ()  [unwired: 1 in, 1 out]
          }
        }
        n90 = call <vilib>:"Add State(s) to Queue__JKI_lib_State_Machine.vi"("State(s) in Front (\"\")"=w206, "State(s) in (\"\")"=w212) -> ("States Out"=w211:string)  [unwired: 13 in]
      }
      frame "TimeSample:TimeSampleStart" {
        # "Your code here.\n(You can make a copy of, or modify, this frame)"
        n91 = Increment(x="时") -> (x+1=w253:u16)
        n92 = Bundle By Name(cluster=w247, "定时采样信息.检测区域"="检测区域", "定时采样信息.时"=w253, "定时采样信息.分钟"="分钟", "定时采样信息.供电位置"="检测位置", "定时采样信息.是否启动"="是否启动", "定时采样信息.备注"="备注", "定时采样信息.电源电压"="电源电压", "定时采样信息.电源频率"="电源频率（Hz）") -> (w256:T4)
        n93 = call <vilib>:"Add State(s) to Queue__JKI_lib_State_Machine.vi"("State(s) in (\"\")"=w259) -> ("States Out"=w258:string)  [unwired: 14 in]
      }
      frame "----------Database---------" {
        # "Your code here.\n(You can make a copy of, or modify, this frame)"
        n94 = call <vilib>:"Add State(s) to Queue__JKI_lib_State_Machine.vi"("State(s) in (\"\")"=w263) -> ("States Out"=w262:string)  [unwired: 14 in]
      }
      frame "Database:LoadAreaName" {
        # "Your code here.\n(You can make a copy of, or modify, this frame)"
        n95 = control-ref of="检测区域"() -> (w268:refnum<vi>)
        n96 = call "GetVandBeishu.vi"() -> ("电压倍数"=w265:string)  [unwired: 9 in, 2 out]
        n97 = call "GetDBAreaName.vi"("ComboBox输入"=w268) -> ("所有记录"=w267:string[])  [unwired: 9 in, 1 out]
        n98 = call "ZhuanVbeishu.vi"("电压倍数"=w265) -> ("电压范围"=w264:string, "最大电压值"=w266:i32)  [unwired: 9 in]
        n99 = Bundle By Name(cluster=w270, "SampleAreaName"=w267, "电源倍数"=w265, "最大电压值"=w266) -> (w269:T4)
        n100 = property on="电压范围" class="Str"("Text.Text"=w264) -> ()  [unwired: 2 in, 2 out]
        n101 = call <vilib>:"Add State(s) to Queue__JKI_lib_State_Machine.vi"("State(s) in (\"\")"=w273) -> ("States Out"=w272:string)  [unwired: 14 in]
      }
    }
  }
